vi "Set Default.vi"(8 "error in (no error)":errorcluster, 11 "Flex Msg in":refnum<class "Flex Msg.lvclass">) -> (0 "error out":errorcluster, 3 "Flex Msg out":refnum<class "Flex Msg.lvclass">)   [LabVIEW 2020, in "Msg.lvlib" / "Flex Msg.lvclass"]
doc: "Restore private data to a defined default state.\n\nDefault implementation does nothing."
uses:
  Flex Msg.lvclass
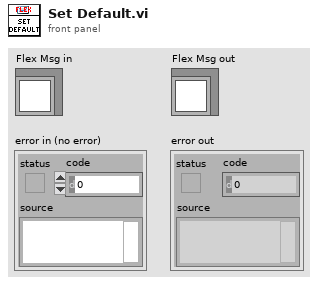
[diagram p1: front panel]
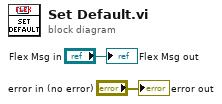
[diagram p0: block diagram]
diagram:
  "error out" <- "error in (no error)"
  "Flex Msg out" <- "Flex Msg in"
